vi "populator.vi"(11 "Temperature Control Parameters":T1 {"End Temp" format="%.2f"; "Temp Step" format="%.2f"; "Start Temp" format="%.2f"}) -> (2 "N temps":i32=6, 3 "Temp Array":dbl[](array[numeric]))   [LabVIEW 2017]
uses:
  P3 R 10-24 to R 10-31/P3 start/typedefs/temp control params.ctl
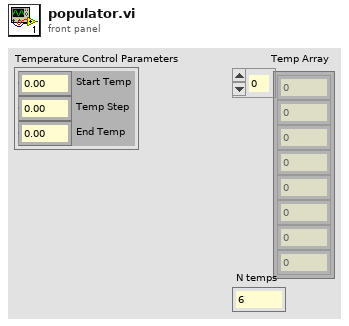
[diagram p1: front panel]
types:
  T1 = typedef "temp control params.ctl" = cluster{"Start Temp":dbl, "Temp Step":dbl, "End Temp":dbl}
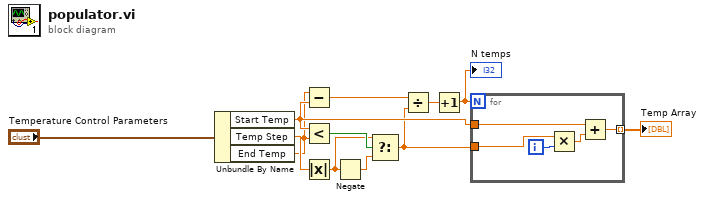
[diagram p0: block diagram]
diagram:
  n1 = Unbundle By Name("Temperature Control Parameters") -> ("Start Temp"=w6:dbl, "Temp Step"=w9:dbl, "End Temp"=w5:dbl)
  n2 = Subtract(x=w5, y=w6) -> (x-y=w11:dbl)
  n3 = Less?(x=w6, y=w5) -> (x < y?=w4:bool)
  n4 = Absolute Value(x=w9) -> (abs(x)=w1:dbl)
  n5 = Negate(x=w1) -> (-x=w2:dbl)
  n6 = Select(t=w1, s=w4, f=w2) -> (s? t:f=w3:dbl)
  n7 = Divide(x=w11, y=w3) -> (x/y=w10:dbl)
  n8 = Increment(x=w10) -> (x+1=w7:dbl)
  "N temps" <- w7
  n9 = for {
    N: w7 -> [_]
    tunnel: w3 -> [w17]
    tunnel: w6 -> [w15]
    tunnel: [w13] -> w8 mode=indexing
    i -> [w16]
    n10 = Multiply(x=w17, y=w16) -> (x*y=w14:dbl)
    n11 = Add(x=w15, y=w14) -> (x+y=w13:dbl)
  }
  "Temp Array" <- w8
